vi "7StateStateMachine.vi"() -> ()   [LabVIEW 2017]
uses:
  Control 1.ctl
panel:
  in  "stop":bool
  out "Enum":T1
  in  "turnAroundToFreestyle?":bool
  in  "approachingElementToFreestyle?":bool
  in  "guidedDriveToFreestyle?":bool
  in  "freestyleToTurnAround?":bool
  in  "freestyleToDriveDistance?":bool
  in  "freestyleToApproachingElement?":bool
  in  "freestyleToTurnAngle?":bool
  in  "freestyleToGuidedDrive?":bool
  in  "turnAngleToDefault?":bool
  in  "turnAngleToFreestyle?":bool
  in  "driveDistanceToTurnAngle?":bool
  in  "driveDistanceToDefault?":bool
  in  "driveDistanceToFreestyle?":bool
  in  "defaultToFreestyle?":bool
  in  "defaultToTurnAngle?":bool
  in  "defaultToDriveDistance?":bool
  # "toDefault?"
  # "toDriveDistance?"
  # "toTurnAngle?"
  # "toFreestyle?"
  # "toGuidedDrive?"
  # "toApproachingElement?"
  # "toTurnAround?"
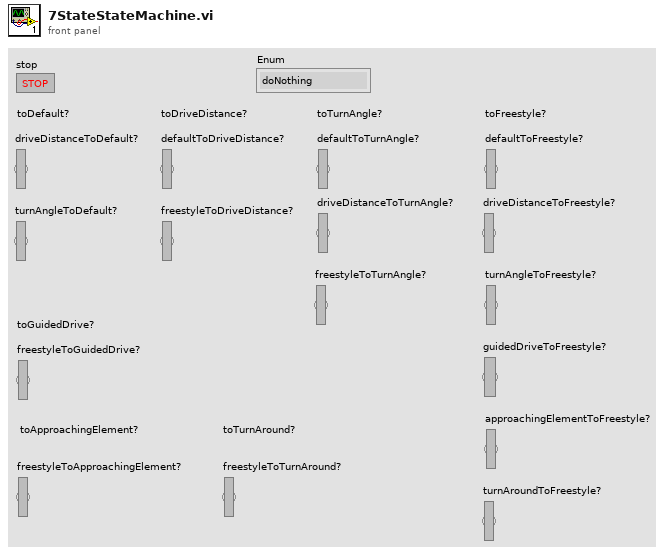
[diagram p1: front panel]
types:
  T1 = typedef "Control 1.ctl" = enum16{"doNothing", "driveDistance", "turnAngle", "freestyle", "guidedDrive", "approachingElement", "turnAround"}
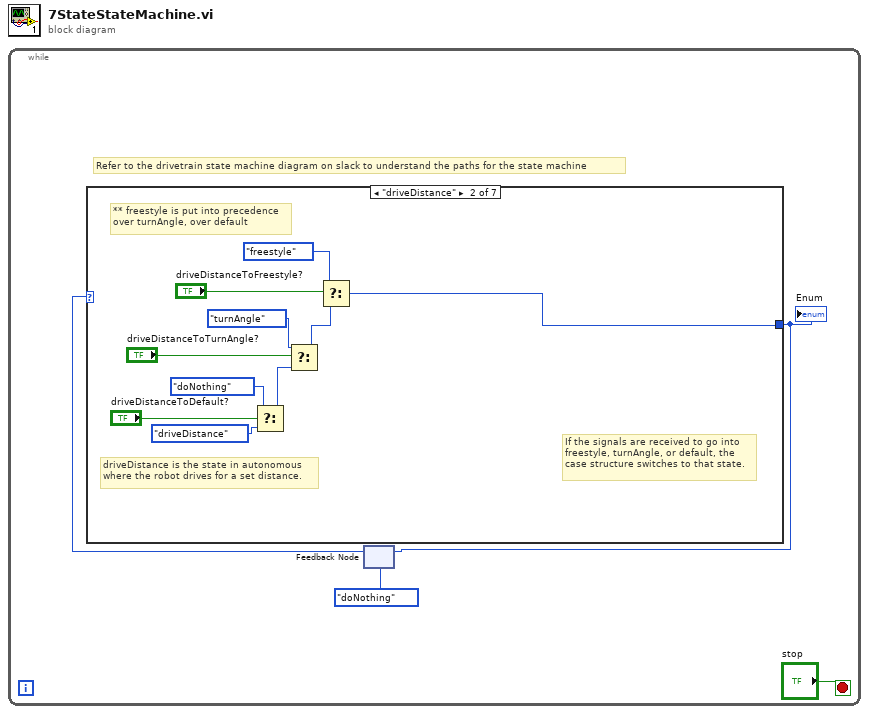
[diagram p0: block diagram]
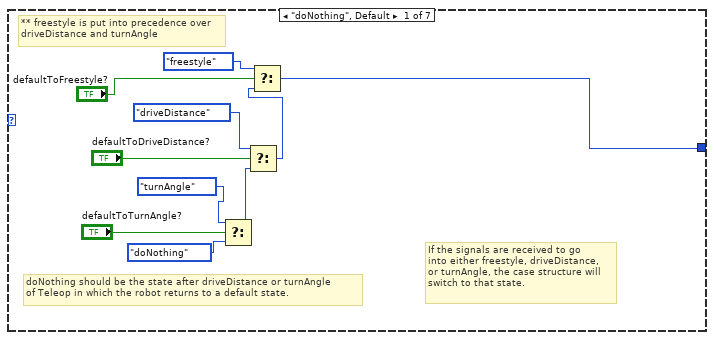
[diagram p2: hidden frame]
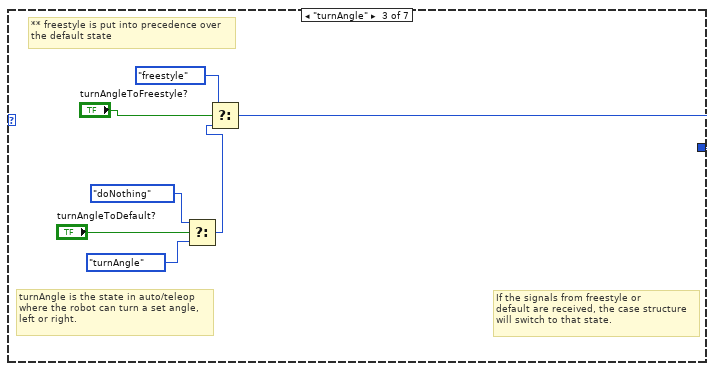
[diagram p3: hidden frame]
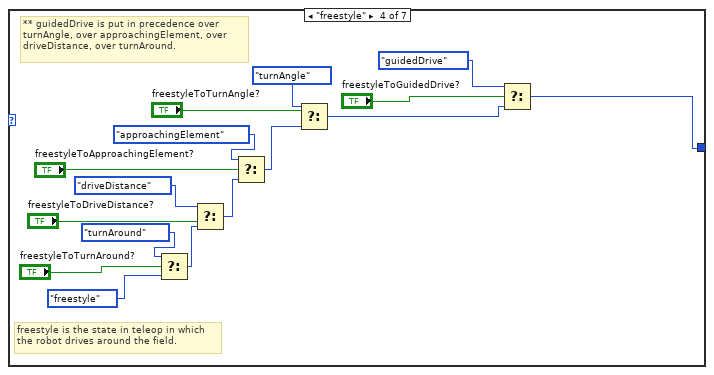
[diagram p4: hidden frame]
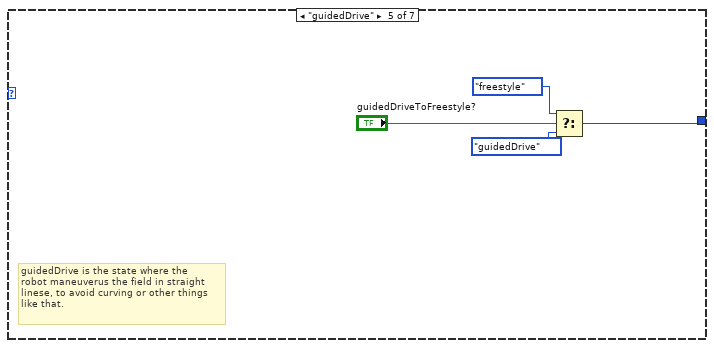
[diagram p5: hidden frame]
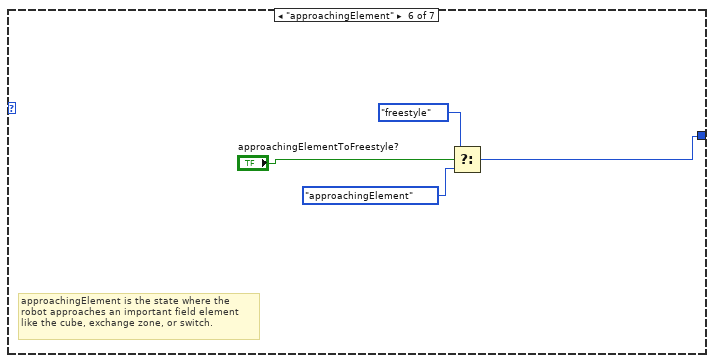
[diagram p6: hidden frame]
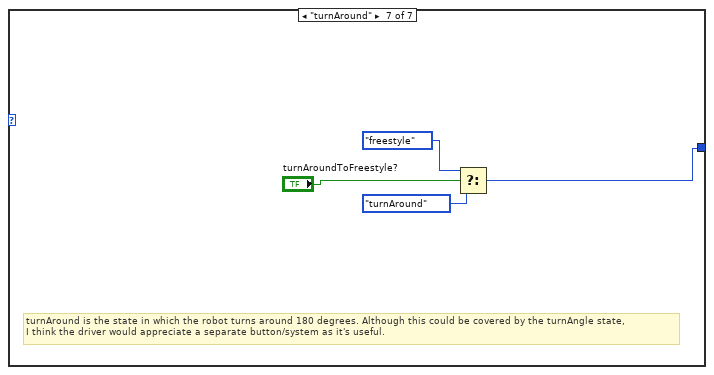
[diagram p7: hidden frame]
diagram:
  n1 = while {
    stop <- "stop" stop-if-true
    # "Refer to the drivetrain state machine diagram on slack to understand the paths for the state machine"
    n2 = feedback #1(Control_1."doNothing") -> (w3:T1)
    n3 = case shown="\"driveDistance\"" w3 {
      tunnel: [w9 w16 w29 w45 w48 w52 w57] -> w2
      frame "doNothing", Default {
        # "** freestyle is put into precedence over\ndriveDistance and turnAngle"
        # "If the signals are received to go\ninto either freestyle, driveDistance,\nor turnAngle, the case structure will\nswitch to that state."
        # "doNothing should be the state after driveDistance or turnAngle \nof Teleop in which the robot returns to a default state."
        n4 = Select(t=Control_1."turnAngle", s="defaultToTurnAngle?", f=Control_1."doNothing") -> (s? t:f=w11:T1)
        n5 = Select(t=Control_1."driveDistance", s="defaultToDriveDistance?", f=w11) -> (s? t:f=w10:T1)
        n6 = Select(t=Control_1."freestyle", s="defaultToFreestyle?", f=w10) -> (s? t:f=w9:T1)
      }
      frame "driveDistance" {
        # "If the signals are received to go into\nfreestyle, turnAngle, or default, the\ncase structure switches to that state."
        # "** freestyle is put into precedence\nover turnAngle, over default"
        # "driveDistance is the state in autonomous\nwhere the robot drives for a set distance."
        n7 = Select(t=Control_1."doNothing", s="driveDistanceToDefault?", f=Control_1."driveDistance") -> (s? t:f=w21:T1)
        n8 = Select(t=Control_1."turnAngle", s="driveDistanceToTurnAngle?", f=w21) -> (s? t:f=w19:T1)
        n9 = Select(t=Control_1."freestyle", s="driveDistanceToFreestyle?", f=w19) -> (s? t:f=w16:T1)
      }
      frame "turnAngle" {
        # "If the signals from freestyle or\ndefault are received, the case structure\nwill switch to that state."
        # "turnAngle is the state in auto/teleop\nwhere the robot can turn a set angle,\nleft or right."
        # "** freestyle is put into precedence over\nthe default state"
        n10 = Select(t=Control_1."doNothing", s="turnAngleToDefault?", f=Control_1."turnAngle") -> (s? t:f=w25:T1)
        n11 = Select(t=Control_1."freestyle", s="turnAngleToFreestyle?", f=w25) -> (s? t:f=w29:T1)
      }
      frame "freestyle" {
        # "freestyle is the state in teleop in which \nthe robot drives around the field."
        # "** guidedDrive is put in precedence over\nturnAngle, over approachingElement, over\ndriveDistance, over turnAround."
        n12 = Select(t=Control_1."turnAround", s="freestyleToTurnAround?", f=Control_1."freestyle") -> (s? t:f=w39:T1)
        n13 = Select(t=Control_1."driveDistance", s="freestyleToDriveDistance?", f=w39) -> (s? t:f=w40:T1)
        n14 = Select(t=Control_1."approachingElement", s="freestyleToApproachingElement?", f=w40) -> (s? t:f=w41:T1)
        n15 = Select(t=Control_1."turnAngle", s="freestyleToTurnAngle?", f=w41) -> (s? t:f=w42:T1)
        n16 = Select(t=Control_1."guidedDrive", s="freestyleToGuidedDrive?", f=w42) -> (s? t:f=w45:T1)
      }
      frame "guidedDrive" {
        # "guidedDrive is the state where the \nrobot maneuverus the field in straight\nlinese, to avoid curving or other things\nlike that."
        n17 = Select(t=Control_1."freestyle", s="guidedDriveToFreestyle?", f=Control_1."guidedDrive") -> (s? t:f=w48:T1)
      }
      frame "approachingElement" {
        # "approachingElement is the state where the \nrobot approaches an important field element\nlike the cube, exchange zone, or switch."
        n18 = Select(t=Control_1."freestyle", s="approachingElementToFreestyle?", f=Control_1."approachingElement") -> (s? t:f=w52:T1)
      }
      frame "turnAround" {
        # "turnAround is the state in which the robot turns around 180 degrees. Although this could be covered by the turnAngle state,\nI think the driver would appreciate a separate button/system as it's useful."
        n19 = Select(t=Control_1."freestyle", s="turnAroundToFreestyle?", f=Control_1."turnAround") -> (s? t:f=w57:T1)
      }
    }
    "Enum" <- w2
    n20 = feedback-in #1(w2) -> ()
  }
